vi "主副屏通信slave.vi"() -> ()   [LabVIEW 2016, in "斯坦道多参数.lvlib"]
uses:
  <vilib>/NI/Modbus Library/API/Wrapper/Create TCP Slave.vi
  <vilib>/NI/Modbus Library/API/slave/Modbus Slave.lvclass
  <vilib>/NI/Modbus Library/API/Wrapper/API Main.lvlib
panel:
  in  "停止":bool
  out "read values":u16[](array[numeric])
  in  "write values":u16[](array[numeric])
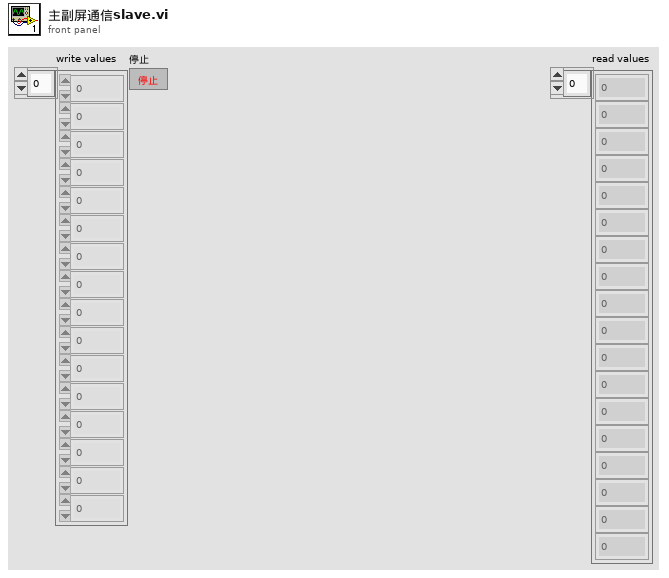
[diagram p1: front panel]
types:
  T1 = cluster{"数据保存间隔":dbl, "水温标样值":dbl, "pH标样值":dbl, "溶解氧标样值":dbl, "电导率标样值":dbl, "浊度标样值":dbl}
  T2 = cluster{"ph":bool, "DO":bool, "Cond":bool, "Turb":bool, "叶绿素a":bool, "藻密度":bool, "ORP":bool}
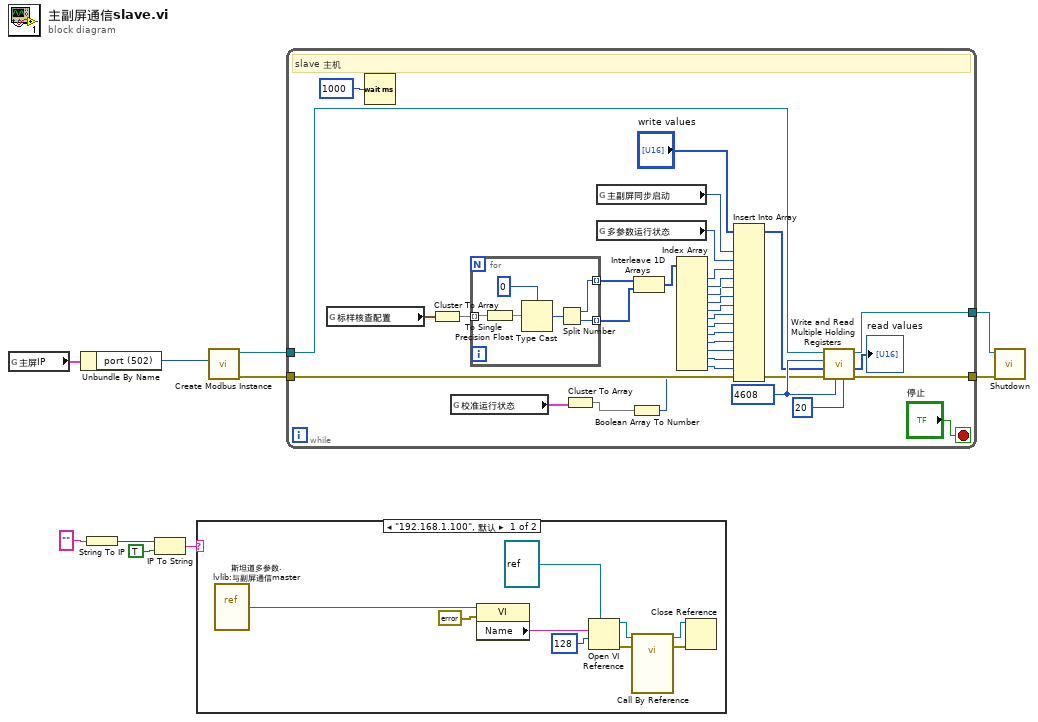
[diagram p0: block diagram]
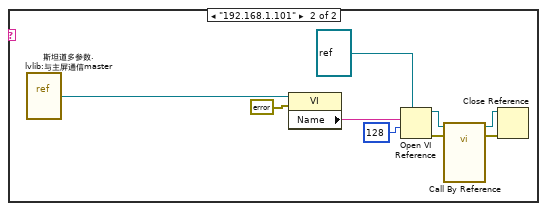
[diagram p2: hidden frame]
diagram:
  n1 = global read "多参数全局变量.vi" "主屏IP"() -> (w6:cluster{"address":string, "port (502)":u16})
  n2 = Unbundle By Name(w6) -> ("port (502)"=w5:u16)
  n3 = String To IP(1:"" ("名称")) -> (0:w4:u32)
  n4 = IP To String(1:TRUE ("句点符号？(F)"), 2:w4) -> (0:w1:string)
  n5 = case shown="\"192.168.1.100\", 默认" w1 {
    frame "192.168.1.100", Default {
      n6 = vi-ref "斯坦道多参数.lvlib:与副屏通信master.vi"() -> (w11:refnum<vi>)
      n7 = property class="VI"(reference=w11, error in=errorcluster {"status"=FALSE, "code"=0, "source"=""} ("错误输出")) -> ("Name"=w12:string)  [unwired: 2 out]
      n8 = Open VI Reference(type specifier VI Refnum (for type only)=refnum<vi> refnum, vi path=w12, options=128 ("选项")) -> (vi reference=w14:refnum<vi>, error out=w16:errorcluster)  [unwired: 3 in]
      n9 = call-by-ref "?"(reference=w14, error in=w16) -> (reference out=w18:refnum<vi>, error out=w17:errorcluster)  [unwired: 12 in]
      n10 = Close Reference(reference=w18, error in (no error)=w17) -> ()  [unwired: 1 out]
    }
    frame "192.168.1.101" {
      n11 = vi-ref "斯坦道多参数.lvlib:与主屏通信master.vi"() -> (w20:refnum<vi>)
      n12 = property class="VI"(reference=w20, error in=errorcluster {"status"=FALSE, "code"=0, "source"=""} ("错误输出")) -> ("Name"=w21:string)  [unwired: 2 out]
      n13 = Open VI Reference(type specifier VI Refnum (for type only)=refnum<vi> refnum, vi path=w21, options=128 ("选项")) -> (vi reference=w23:refnum<vi>, error out=w25:errorcluster)  [unwired: 3 in]
      n14 = call-by-ref "?"(reference=w23, error in=w25) -> (reference out=w27:refnum<vi>, error out=w26:errorcluster)  [unwired: 12 in]
      n15 = Close Reference(reference=w27, error in (no error)=w26) -> ()  [unwired: 1 out]
    }
  }
  n16 = call-poly <vilib>:"Create Modbus Instance.vi"("port (502)"=w5) -> ("error out"=w7:errorcluster, "TCP slave instance"=w10:refnum<class "Modbus Slave.lvclass">)  [unwired: 9 in]
  n17 = while {
    tunnel: w10 -> [w53]
    tunnel: [w58] -> w9
    tunnel: [w57] -> w8
    tunnel: w7 -> [w56]
    stop <- "停止" stop-if-true
    w61 = u16 4608 ("write starting address")
    # "slave 主机"
    n18 = global read "断电保存变量.vi" "标样核查配置"() -> (w48:T1)
    n19 = Wait (ms)(milliseconds to wait=u32 1000 ("等待时间（毫秒）")) -> ()  [unwired: 1 out]
    n20 = Cluster To Array(cluster=w48) -> (array=w47:dbl[])
    n21 = global read "多参数全局变量.vi" "校准运行状态"() -> (w31:T2)
    n22 = for {
      tunnel: w47 -> [w63] mode=indexing
      tunnel: [w65] -> w46 mode=indexing
      tunnel: [w64] -> w45 mode=indexing
      n23 = To Single Precision Float(number=w63) -> (single precision float=w62:sgl)
      n24 = Type Cast(type=0, x=w62) -> (*(type *) &x=w66:i32)
      n25 = Split Number(x=w66) -> (hi(x)=w65:u16, lo(x)=w64:u16)
    }
    n26 = Cluster To Array(cluster=w31) -> (array=w30:bool[])
    n27 = global read "多参数全局变量.vi" "主副屏同步启动"() -> (w50:u16)
    n28 = global read "多参数全局变量.vi" "多参数运行状态"() -> (w49:u16)
    n29 = Boolean Array To Number(Boolean array=w30) -> (number=w29:u32)
    n30 = Interleave 1D Arrays(w46, w45) -> (w44:u16[])
    n31 = Index Array(array=w44) -> (element #1=w43:u16, element #2=w42:u16, element #3=w41:u16, element #4=w40:u16, element #5=w39:u16, element #6=w38:u16, element #7=w37:u16, element #8=w36:u16, element #9=w35:u16, element #10=w34:u16, element #11=w33:u16, element #12=w32:u16)  [unwired: 12 in]
    n32 = Insert Into Array(array="write values", new element #1=w50, new element #2=w49, new element #3=w43, new element #4=w42, new element #5=w41, new element #6=w40, new element #7=w39, new element #8=w38, new element #9=w37, new element #10=w36, new element #11=w35, new element #12=w34, new element #13=w33, new element #14=w32, new element #15=w29) -> (w51:u16[])  [unwired: 1 in]
    n33 = call-dynamic "Write and Read Multiple Holding Registers.vi"("read count"=u16 20, "read starting address"=w61, "error in"=w56, "write values"=w51, "write starting address"=w61, "Modbus instance in"=w53) -> ("error out"=w57:errorcluster, "read values"=→"read values":u16[], "Modbus instance out"=w58:refnum<class "Modbus Slave.lvclass">)  [unwired: 3 in]
  }
  n34 = call-dynamic "Shutdown.vi"("error in"=w8, "Modbus slave in"=w9) -> ()  [unwired: 9 in, 1 out]
